vi "Merge Sort 2D String Arrays.vi"(0 "2D String Array A":string[][](array[string]), 1 "Ignore Duplicates? (F)":bool=TRUE, 3 "2D String Array B":string[][](array[string])) -> (6 "Sorted 2D String Array":string[][](array[string]))   [LabVIEW 2013]
panel:
  out "A Index":i32
  out "B Index":i32
  out "B Count":i32
  out "A Count":i32
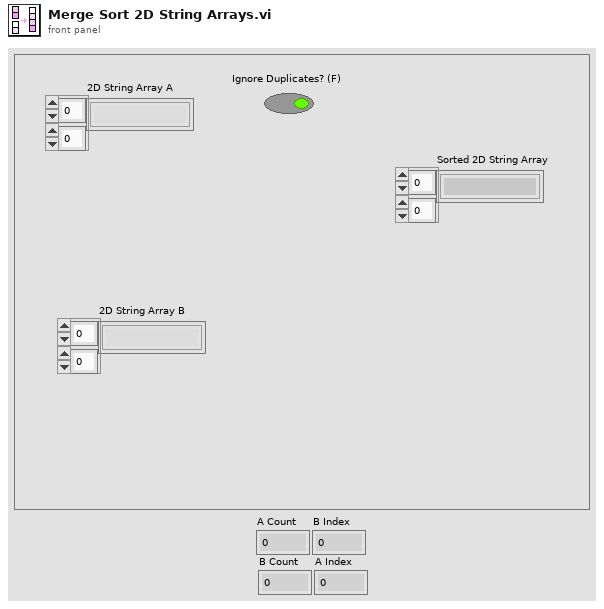
[diagram p1: front panel]
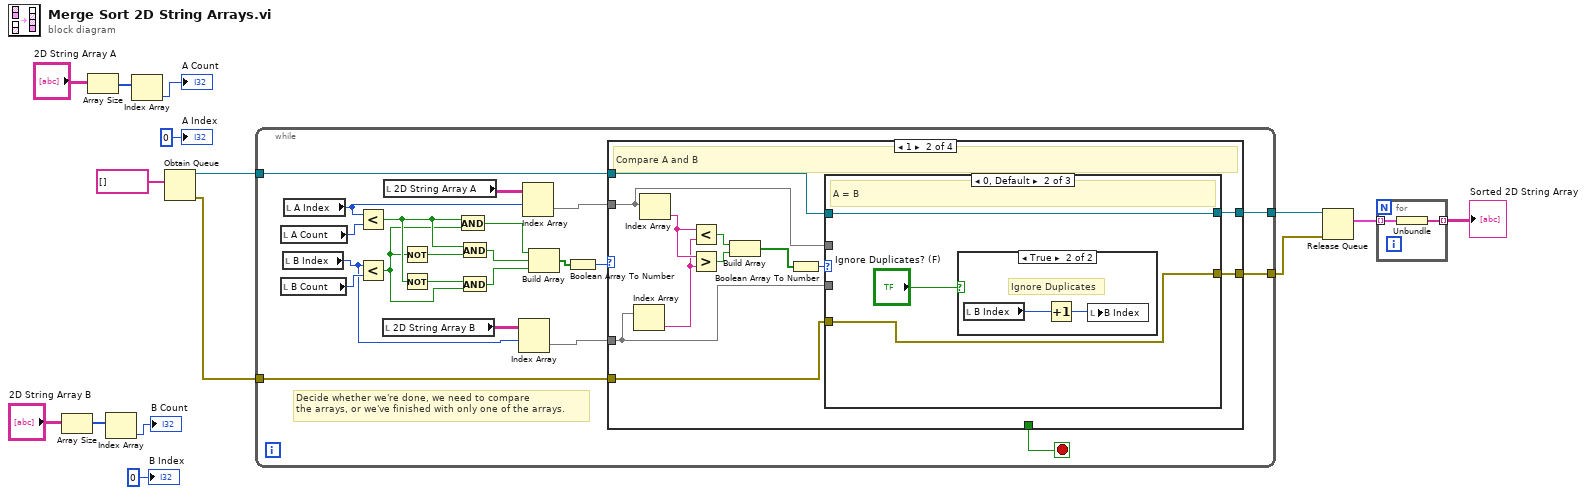
[diagram p0: block diagram]
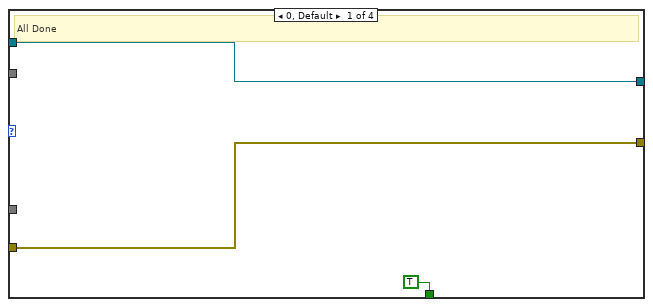
[diagram p2: hidden frame]
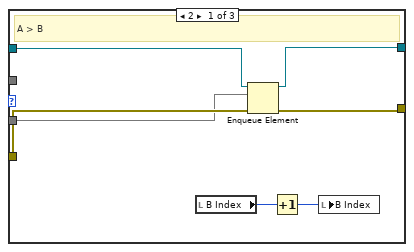
[diagram p3: hidden frame]
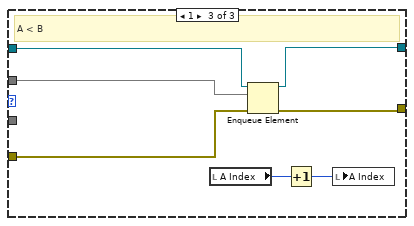
[diagram p5: hidden frame]
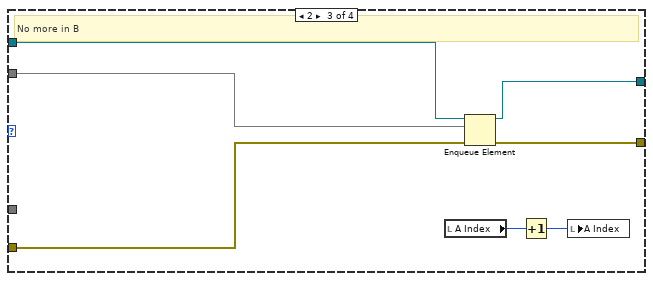
[diagram p6: hidden frame]
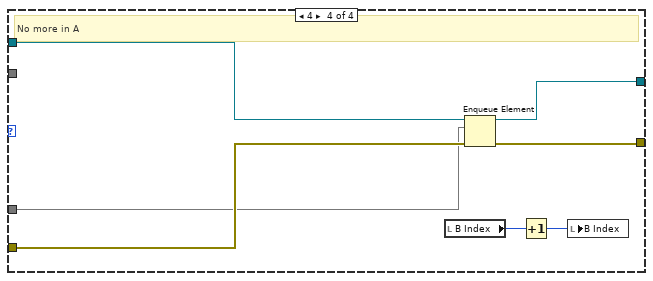
[diagram p7: hidden frame]
diagram:
  n1 = Array Size(array="2D String Array B") -> (size(s)=w4:i32[])
  n2 = Array Size(array="2D String Array A") -> (size(s)=w6:i32[])
  n3 = Index Array(array=w4) -> (element=→"B Count":i32)  [unwired: 1 in]
  n4 = Index Array(array=w6) -> (element=→"A Count":i32)  [unwired: 1 in]
  n5 = Obtain Queue(element data type=string[] []) -> (queue out=w14:refnum<queue>, error out=w13:errorcluster)  [unwired: 4 in, 1 out]
  n6 = while {
    tunnel: w14 -> [w26]
    tunnel: [w25] -> w8
    tunnel: [w24] -> w15
    tunnel: w13 -> [w23]
    stop <- w16 stop-if-true
    # "Decide whether we're done, we need to compare\nthe arrays, or we've finished with only one of the arrays."
    n7 = local read "A Count"() -> (w37:i32)
    n8 = local read "B Count"() -> (w36:i32)
    n9 = local read "B Index"() -> (w19:i32)
    n10 = local read "A Index"() -> (w21:i32)
    n11 = Less?(x=w21, y=w37) -> (x < y?=w33:bool)
    n12 = Less?(x=w19, y=w36) -> (x < y?=w32:bool)
    n13 = local read "2D String Array B"() -> (w20:string[][])
    n14 = local read "2D String Array A"() -> (w22:string[][])
    n15 = Not(x=w32) -> (.not. x?=w30:bool)
    n16 = Not(x=w33) -> (.not. x?=w29:bool)
    n17 = And(x=w33, y=w32) -> (x .and. y?=w35:bool)
    n18 = And(x=w33, y=w30) -> (x .and. y?=w34:bool)
    n19 = And(x=w29, y=w32) -> (x .and. y?=w31:bool)
    n20 = Index Array(array=w20, index (row)=w19) -> (element=w18:string[])  [unwired: 1 in]
    n21 = Index Array(array=w22, index (row)=w21) -> (element=w17:string[])  [unwired: 1 in]
    n22 = Build Array(w35, w34, w31) -> (w28:bool[])
    n23 = Boolean Array To Number(Boolean array=w28) -> (number=w27:u32)
    n24 = case shown="1" w27 {
      tunnel: w26 -> [w40 w52 w78 w85]
      tunnel: w17 -> [_ w44 w76 _]
      tunnel: w18 -> [_ w42 _ w83]
      tunnel: w23 -> [w39 w45 w77 w84]
      tunnel: [w39 w51 w74 w81] -> w25
      tunnel: [w40 w50 w75 w82] -> w24
      tunnel: [TRUE _ _ _] -> w16
      frame 0, Default {
        # "All Done"
      }
      frame 1 {
        # "Compare A and B"
        n25 = Index Array(array=w42) -> (element=w41:string)  [unwired: 1 in]
        n26 = Index Array(array=w44) -> (element=w43:string)  [unwired: 1 in]
        n27 = Less?(x=w43, y=w41) -> (x < y?=w49:bool)
        n28 = Greater?(x=w43, y=w41) -> (0:w48:bool)
        n29 = Build Array(w49, w48) -> (w47:bool[])
        n30 = Boolean Array To Number(Boolean array=w47) -> (number=w46:u32)
        n31 = case shown="0, Default" w46 {
          tunnel: w52 -> [w59 w60 w71]
          tunnel: w44 -> [_ _ w70]
          tunnel: w42 -> [w53 _ _]
          tunnel: w45 -> [w58 w61 w69]
          tunnel: [w56 w61 w67] -> w51
          tunnel: [w57 w60 w68] -> w50
          frame 2 {
            # "A > B"
            n32 = local read "B Index"() -> (w54:i32)
            n33 = Enqueue Element(queue=w59, element=w53, error in (no error)=w58) -> (queue out=w57:refnum<queue>, error out=w56:errorcluster)  [unwired: 1 in, 1 out]
            n34 = Increment(x=w54) -> (x+1=w55:i32)
            n35 = local write "B Index"(w55) -> ()
          }
          frame 0, Default {
            # "A = B"
            n36 = case shown="True" "Ignore Duplicates? (F)" {
              frame False {
              }
              frame True {
                # "Ignore Duplicates"
                n37 = local read "B Index"() -> (w64:i32)
                n38 = Increment(x=w64) -> (x+1=w63:i32)
                n39 = local write "B Index"(w63) -> ()
              }
            }
          }
          frame 1 {
            # "A < B"
            n40 = local read "A Index"() -> (w65:i32)
            n41 = Enqueue Element(queue=w71, element=w70, error in (no error)=w69) -> (queue out=w68:refnum<queue>, error out=w67:errorcluster)  [unwired: 1 in, 1 out]
            n42 = Increment(x=w65) -> (x+1=w66:i32)
            n43 = local write "A Index"(w66) -> ()
          }
        }
      }
      frame 2 {
        # "No more in B"
        n44 = local read "A Index"() -> (w72:i32)
        n45 = Enqueue Element(queue=w78, element=w76, error in (no error)=w77) -> (queue out=w75:refnum<queue>, error out=w74:errorcluster)  [unwired: 1 in, 1 out]
        n46 = Increment(x=w72) -> (x+1=w73:i32)
        n47 = local write "A Index"(w73) -> ()
      }
      frame 4 {
        # "No more in A"
        n48 = local read "B Index"() -> (w79:i32)
        n49 = Enqueue Element(queue=w85, element=w83, error in (no error)=w84) -> (queue out=w82:refnum<queue>, error out=w81:errorcluster)  [unwired: 1 in, 1 out]
        n50 = Increment(x=w79) -> (x+1=w80:i32)
        n51 = local write "B Index"(w80) -> ()
      }
    }
  }
  n52 = Release Queue(queue=w15, error in (no error)=w8) -> (remaining elements=w2:cluster{string[]}[])  [unwired: 1 in, 2 out]
  n53 = for {
    tunnel: w2 -> [w87] mode=indexing
    tunnel: [w86] -> w1 mode=indexing
    n54 = Unbundle(w87) -> (w86:string[])
  }
  "Sorted 2D String Array" <- w1
  "A Index" <- 0 ("A Index")
  "B Index" <- 0 ("B Index")
